vi "save_to_binary_file.vi"(4 "offset (0)":dbl, 5 "prepend array size?":bool, 6 "multiplication factor (1)":dbl=1.0, 7 "force format?":T1, 8 "error in (no error)":errorcluster, 9 "byte order (0:big-endian, network order)":T2(ring)=enum."little-endian", 10 "Path":path, 11 "Image in":refnum<class "Image.lvclass">) -> (0 "error out":errorcluster, 3 "Image out":refnum<class "Image.lvclass">)   [LabVIEW 2010, in "Image.lvclass"]
uses:
  Image.lvclass
  target_format_enum.ctl
  storage_mode.ctl
  error_codes_ring.ctl
  ErrorController/ErrorController/class_data.vi
  ErrorController/ErrorController/ErrorController.lvclass
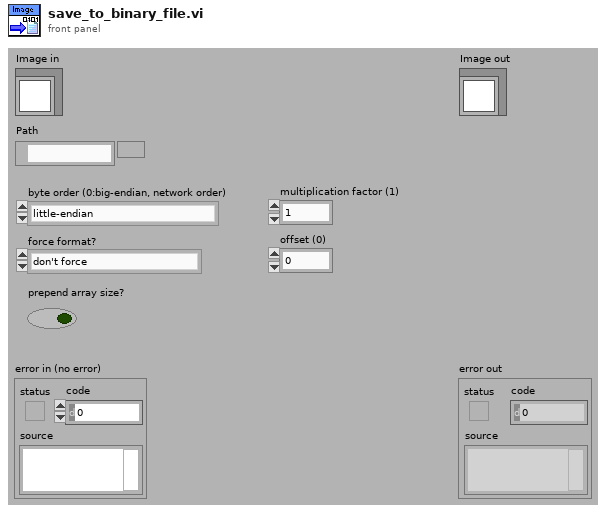
[diagram p1: front panel]
types:
  T1 = typedef "target_format_enum.ctl" = enum16{"don't force", "uint8", "uint16", "int16", "uint32", "int32", "single float"}
  T2 = enum16{"big-endian, network order", "native, host order", "little-endian"}
  T3 = typedef "Image.lvclass/storage_mode.ctl" = enum16{"RAM", "disk"}
  T4 = typedef "Image Type" = u32
  T5 = typedef "IMAQ Image.ctl" = refnum<image>
  T6 = typedef "Color (U64)" = cluster{"Plane 3 (Blue)":u16, "Plane 2 (Green)":u16, "Plane 1 (Red)":u16, "Plane 4 (alpha)":u16}
  T7 = typedef "Image.lvclass/error_codes_ring.ctl" = u16
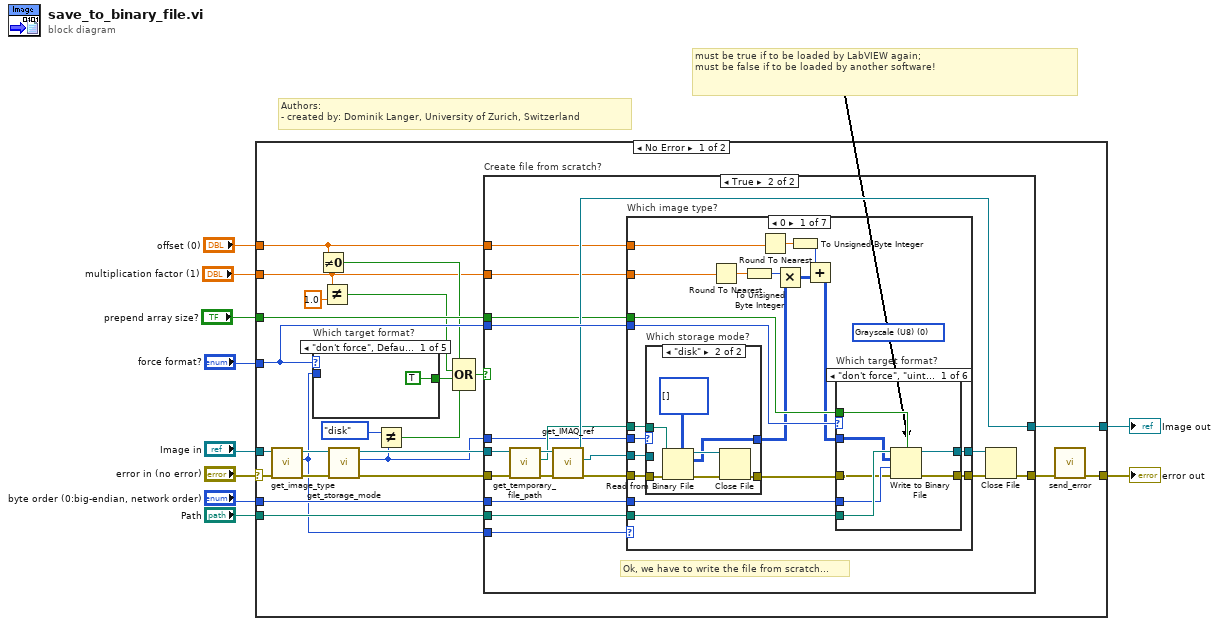
[diagram p0: block diagram]
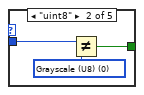
[diagram p2: hidden frame]
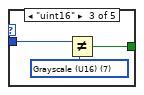
[diagram p3: hidden frame]
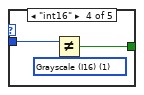
[diagram p4: hidden frame]
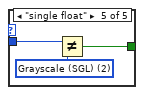
[diagram p5: hidden frame]
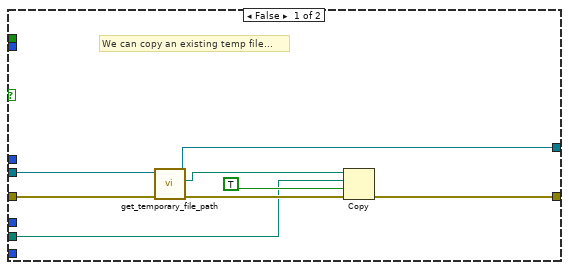
[diagram p6: hidden frame]
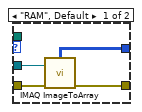
[diagram p7: hidden frame]
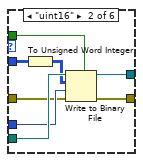
[diagram p8: hidden frame]
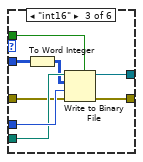
[diagram p9: hidden frame]
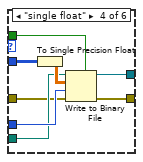
[diagram p10: hidden frame]
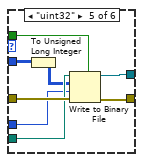
[diagram p11: hidden frame]
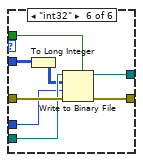
[diagram p12: hidden frame]
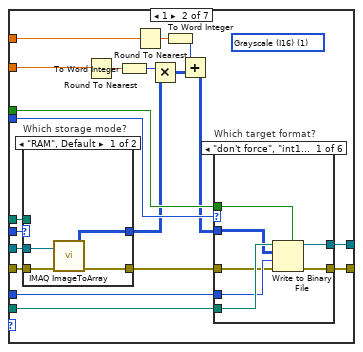
[diagram p13: hidden frame]
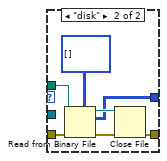
[diagram p14: hidden frame]
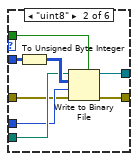
[diagram p15: hidden frame]
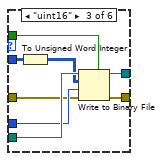
[diagram p16: hidden frame]
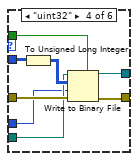
[diagram p17: hidden frame]
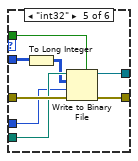
[diagram p18: hidden frame]
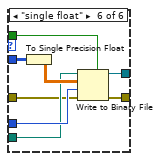
[diagram p19: hidden frame]
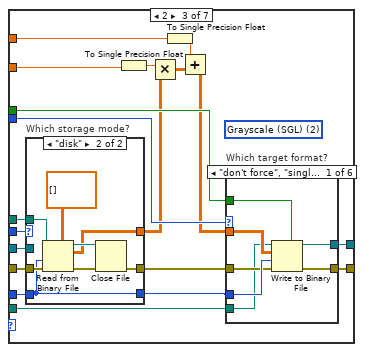
[diagram p20: hidden frame]
diagram:
  # "must be true if to be loaded by LabVIEW again;\nmust be false if to be loaded by another software!"
  # "Authors: \n- created by: Dominik Langer, University of Zurich, Switzerland"
  n1 = case shown="No Error" "error in (no error)" {
    selector: "error in (no error)" -> [w34 w414]
    tunnel: [w12 w414] -> w5
    tunnel: [w25 w413] -> w4
    tunnel: "Image in" -> [w33 w413]
    tunnel: "Path" -> [w26 _]
    tunnel: "byte order (0:big-endian, network order)" -> [w27 _]
    tunnel: "force format?" -> [w23 _]
    tunnel: "prepend array size?" -> [w22 _]
    tunnel: "offset (0)" -> [w14 _]
    tunnel: "multiplication factor (1)" -> [w13 _]
    frame No Error {
      n2 = call-dynamic "get_image_type.vi"("error in (no error)"=w34, "Image.lvclass in"=w33) -> ("error out"=w32:errorcluster, "Image Type"=w24:T4, "Image.lvclass out"=w31:refnum<class "Image.lvclass">)  [unwired: 6 in, 1 out]
      n3 = case "Which target format?" shown="\"don't force\", Default" w23 {
        tunnel: w24 -> [_ w38 w41 w44 w47]
        tunnel: [TRUE w36 w39 w42 w45] -> w16
        frame "don't force", Default {
        }
        frame "uint8" {
          w37 = T4 0 items=["Grayscale (U8)", "Grayscale (I16)", "Grayscale (SGL)", "Complex (CSG)", "RGB (U32)", "HSL (U32)", "RGB (U64)", "Grayscale (U16)"] ("y")
          n4 = Not Equal?(x=w38, y=w37) -> (x != y?=w36:bool)
        }
        frame "uint16" {
          w40 = T4 7 items=["Grayscale (U8)", "Grayscale (I16)", "Grayscale (SGL)", "Complex (CSG)", "RGB (U32)", "HSL (U32)", "RGB (U64)", "Grayscale (U16)"] ("y")
          n5 = Not Equal?(x=w41, y=w40) -> (x != y?=w39:bool)
        }
        frame "int16" {
          w43 = T4 1 items=["Grayscale (U8)", "Grayscale (I16)", "Grayscale (SGL)", "Complex (CSG)", "RGB (U32)", "HSL (U32)", "RGB (U64)", "Grayscale (U16)"] ("y")
          n6 = Not Equal?(x=w44, y=w43) -> (x != y?=w42:bool)
        }
        frame "single float" {
          w46 = T4 2 items=["Grayscale (U8)", "Grayscale (I16)", "Grayscale (SGL)", "Complex (CSG)", "RGB (U32)", "HSL (U32)", "RGB (U64)", "Grayscale (U16)"] ("y")
          n7 = Not Equal?(x=w47, y=w46) -> (x != y?=w45:bool)
        }
      }
      n8 = Not Equal To 0?(x=w14) -> (x != 0?=w20:bool)
      n9 = Not Equal?(x=w13, y=1.0) -> (x != y?=w15:bool)
      n10 = call-dynamic "get_storage_mode.vi"("error in (no error)"=w32, "Image.lvclass in"=w31) -> ("error out"=w29:errorcluster, "storage mode"=w19:T3, "Image.lvclass out"=w28:refnum<class "Image.lvclass">)  [unwired: 7 out]
      n11 = Not Equal?(x=storage_mode."disk", y=w19) -> (x != y?=w18:bool)
      n12 = Compound Arithmetic op=OR(w20, w15, w16, w18) -> (w17:bool)
      n13 = case "Create file from scratch?" shown="True" w17 {
        tunnel: w29 -> [w52 w66]
        tunnel: [w51 w62] -> w11
        tunnel: w28 -> [w49 w65]
        tunnel: w27 -> [_ w70]
        tunnel: w26 -> [w50 w69]
        tunnel: [w48 w61] -> w25
        tunnel: w24 -> [_ w68]
        tunnel: w23 -> [_ w67]
        tunnel: w22 -> [_ w59]
        tunnel: w19 -> [_ w58]
        tunnel: w14 -> [_ w57]
        tunnel: w13 -> [_ w56]
        frame False {
          # "We can copy an existing temp file..."
          n14 = call-dynamic "get_temporary_file_path.vi"("error in (no error)"=w52, "Image.lvclass in"=w49) -> ("error out"=w55:errorcluster, "temporary file path"=w54:path, "Image.lvclass out"=w48:refnum<class "Image.lvclass">)  [unwired: 7 out]
          n15 = Copy(8:w55, 9:TRUE ("overwrite (F)"), 10:w50, 11:w54) -> (0:w51:errorcluster)  [unwired: 3 out]
        }
        frame True {
          # "Ok, we have to write the file from scratch..."
          n16 = call-dynamic "get_temporary_file_path.vi"("error in (no error)"=w66, "Image.lvclass in"=w65) -> ("error out"=w64:errorcluster, "temporary file path"=w60:path, "Image.lvclass out"=w63:refnum<class "Image.lvclass">)  [unwired: 7 out]
          n17 = call-dynamic "get_IMAQ_ref.vi"("error in (no error)"=w64, "Image.lvclass in"=w63) -> ("error out"=w74:errorcluster, "Image"=w73:T5, "Image.lvclass out"=w61:refnum<class "Image.lvclass">)  [unwired: 7 out]
          n18 = case "Which image type?" shown="0" w68 {
            tunnel: [w94 w172 w245 w315 w325 w347 w406] -> w72
            tunnel: w73 -> [w87 w164 w248 w317 w324 w339 _]
            tunnel: w74 -> [w89 w167 w249 w318 w326 w342 w407]
            tunnel: [w93 w171 w244 w313 w322 w346 _] -> w71
            tunnel: w69 -> [w92 w169 w246 w312 w321 w343 _]
            tunnel: w70 -> [w91 w170 w241 w311 w320 w344 _]
            tunnel: w67 -> [w90 w168 w243 _ _ w345 _]
            tunnel: w60 -> [w86 w165 w242 _ _ w340 _]
            tunnel: w59 -> [w85 w163 w239 w310 w319 w338 _]
            tunnel: w58 -> [w84 w162 w238 _ _ w337 _]
            tunnel: w57 -> [w77 w158 w231 _ _ w331 _]
            tunnel: w56 -> [w78 w160 w234 _ _ w332 _]
            frame 0 {
              (unwired) T4 0 items=["Grayscale (U8)", "Grayscale (I16)", "Grayscale (SGL)", "Complex (CSG)", "RGB (U32)", "HSL (U32)", "RGB (U64)", "Grayscale (U16)"] ("Image Type")
              n19 = case "Which storage mode?" shown="\"disk\"" w84 {
                tunnel: w89 -> [w98 w103]
                tunnel: w87 -> [w97 _]
                tunnel: [w96 w102] -> w88
                tunnel: [w95 w100] -> w75
                tunnel: w86 -> [_ w101]
                frame "RAM", Default {
                  n20 = call "IMAQ ImageToArray"("error in (no error)"=w98, "Image"=w97) -> ("error out"=w96:errorcluster, "Image Pixels (U8)"=w95:u8[][])  [unwired: 1 in, 4 out]
                }
                frame "disk" {
                  n21 = Read from Binary File(5:u8[][] [], 8:w103, 11:w101) -> (0:w105:errorcluster, 2:w100:u8[][], 3:w104:refnum<file>)  [unwired: 1 in, 3 out]
                  n22 = Close File(refnum=w104, error in=w105) -> (error out=w102:errorcluster)  [unwired: 1 out]
                }
              }
              n23 = Round To Nearest(number=w78) -> (nearest integer value=w82:dbl)
              n24 = To Unsigned Byte Integer(number=w82) -> (unsigned 8bit integer=w83:u8)
              n25 = Round To Nearest(number=w77) -> (nearest integer value=w81:dbl)
              n26 = Multiply(x=w83, y=w75) -> (x*y=w79:u8[][])
              n27 = To Unsigned Byte Integer(number=w81) -> (unsigned 8bit integer=w80:u8)
              n28 = Add(x=w80, y=w79) -> (x+y=w76:u8[][])
              n29 = case "Which target format?" shown="\"don't force\", \"uint8\", Default" w90 {
                tunnel: [w112 w117 w128 w135 w139 w151] -> w94
                tunnel: w88 -> [w107 w114 w123 w130 w144 w152]
                tunnel: [w111 w116 w125 w134 w138 w150] -> w93
                tunnel: w92 -> [w110 w120 w126 w132 w141 w147]
                tunnel: w91 -> [w109 w119 w127 w133 w140 w146]
                tunnel: w76 -> [w108 w115 w122 w131 w143 w149]
                tunnel: w85 -> [w106 w113 w121 w129 w142 w148]
                frame "don't force", "uint8", Default {
                  n30 = Write to Binary File(file (use dialog)=w110, data=w108, error in=w107, 5:w106, 9:w109) -> (refnum out=w111:refnum<file>, error out=w112:errorcluster)  [unwired: 2 out]
                }
                frame "uint16" {
                  n31 = To Unsigned Word Integer(number=w115) -> (unsigned 16bit integer=w118:u16[][])
                  n32 = Write to Binary File(file (use dialog)=w120, data=w118, error in=w114, 5:w113, 9:w119) -> (refnum out=w116:refnum<file>, error out=w117:errorcluster)  [unwired: 2 out]
                }
                frame "int16" {
                  n33 = To Word Integer(number=w122) -> (16bit integer=w124:i16[][])
                  n34 = Write to Binary File(file (use dialog)=w126, data=w124, error in=w123, 5:w121, 9:w127) -> (refnum out=w125:refnum<file>, error out=w128:errorcluster)  [unwired: 2 out]
                }
                frame "single float" {
                  n35 = To Single Precision Float(number=w131) -> (single precision float=w136:sgl[][])
                  n36 = Write to Binary File(file (use dialog)=w132, data=w136, error in=w130, 5:w129, 9:w133) -> (refnum out=w134:refnum<file>, error out=w135:errorcluster)  [unwired: 2 out]
                }
                frame "uint32" {
                  n37 = To Unsigned Long Integer(number=w143) -> (unsigned 32bit integer=w137:u32[][])
                  n38 = Write to Binary File(file (use dialog)=w141, data=w137, error in=w144, 5:w142, 9:w140) -> (refnum out=w138:refnum<file>, error out=w139:errorcluster)  [unwired: 2 out]
                }
                frame "int32" {
                  n39 = To Long Integer(number=w149) -> (32bit integer=w145:i32[][])
                  n40 = Write to Binary File(file (use dialog)=w147, data=w145, error in=w152, 5:w148, 9:w146) -> (refnum out=w150:refnum<file>, error out=w151:errorcluster)  [unwired: 2 out]
                }
              }
            }
            frame 1 {
              (unwired) T4 1 items=["Grayscale (U8)", "Grayscale (I16)", "Grayscale (SGL)", "Complex (CSG)", "RGB (U32)", "HSL (U32)", "RGB (U64)", "Grayscale (U16)"] ("Image Type")
              n41 = case "Which storage mode?" shown="\"RAM\", Default" w162 {
                tunnel: w167 -> [w176 w181]
                tunnel: w164 -> [w175 _]
                tunnel: [w174 w180] -> w166
                tunnel: [w173 w178] -> w153
                tunnel: w165 -> [_ w179]
                frame "RAM", Default {
                  n42 = call "IMAQ ImageToArray"("error in (no error)"=w176, "Image"=w175) -> ("error out"=w174:errorcluster, "Image Pixels (I16)"=w173:i16[][])  [unwired: 1 in, 4 out]
                }
                frame "disk" {
                  n43 = Read from Binary File(5:i16[][] [], 8:w181, 11:w179) -> (0:w183:errorcluster, 2:w178:i16[][], 3:w182:refnum<file>)  [unwired: 1 in, 3 out]
                  n44 = Close File(refnum=w182, error in=w183) -> (error out=w180:errorcluster)  [unwired: 1 out]
                }
              }
              n45 = Round To Nearest(number=w160) -> (nearest integer value=w159:dbl)
              n46 = To Word Integer(number=w159) -> (16bit integer=w161:i16)
              n47 = Round To Nearest(number=w158) -> (nearest integer value=w157:dbl)
              n48 = Multiply(x=w161, y=w153) -> (x*y=w155:i16[][])
              n49 = To Word Integer(number=w157) -> (16bit integer=w156:i16)
              n50 = Add(x=w156, y=w155) -> (x+y=w154:i16[][])
              n51 = case "Which target format?" shown="\"don't force\", \"int16\", Default" w168 {
                tunnel: [w190 w197 w203 w213 w221 w229] -> w172
                tunnel: w166 -> [w186 w193 w201 w214 w222 w225]
                tunnel: [w189 w196 w202 w212 w220 w228] -> w171
                tunnel: w169 -> [w188 w195 w206 w208 w218 w226]
                tunnel: w170 -> [w187 w194 w205 w207 w217 w227]
                tunnel: w154 -> [w185 w192 w200 w210 w215 w224]
                tunnel: w163 -> [w184 w191 w199 w209 w219 w223]
                frame "don't force", "int16", Default {
                  n52 = Write to Binary File(file (use dialog)=w188, data=w185, error in=w186, 5:w184, 9:w187) -> (refnum out=w189:refnum<file>, error out=w190:errorcluster)  [unwired: 2 out]
                }
                frame "uint8" {
                  n53 = To Unsigned Byte Integer(number=w192) -> (unsigned 8bit integer=w198:u8[][])
                  n54 = Write to Binary File(file (use dialog)=w195, data=w198, error in=w193, 5:w191, 9:w194) -> (refnum out=w196:refnum<file>, error out=w197:errorcluster)  [unwired: 2 out]
                }
                frame "uint16" {
                  n55 = To Unsigned Word Integer(number=w200) -> (unsigned 16bit integer=w204:u16[][])
                  n56 = Write to Binary File(file (use dialog)=w206, data=w204, error in=w201, 5:w199, 9:w205) -> (refnum out=w202:refnum<file>, error out=w203:errorcluster)  [unwired: 2 out]
                }
                frame "uint32" {
                  n57 = To Unsigned Long Integer(number=w210) -> (unsigned 32bit integer=w211:u32[][])
                  n58 = Write to Binary File(file (use dialog)=w208, data=w211, error in=w214, 5:w209, 9:w207) -> (refnum out=w212:refnum<file>, error out=w213:errorcluster)  [unwired: 2 out]
                }
                frame "int32" {
                  n59 = To Long Integer(number=w215) -> (32bit integer=w216:i32[][])
                  n60 = Write to Binary File(file (use dialog)=w218, data=w216, error in=w222, 5:w219, 9:w217) -> (refnum out=w220:refnum<file>, error out=w221:errorcluster)  [unwired: 2 out]
                }
                frame "single float" {
                  n61 = To Single Precision Float(number=w224) -> (single precision float=w230:sgl[][])
                  n62 = Write to Binary File(file (use dialog)=w226, data=w230, error in=w225, 5:w223, 9:w227) -> (refnum out=w228:refnum<file>, error out=w229:errorcluster)  [unwired: 2 out]
                }
              }
            }
            frame 2 {
              (unwired) T4 2 items=["Grayscale (U8)", "Grayscale (I16)", "Grayscale (SGL)", "Complex (CSG)", "RGB (U32)", "HSL (U32)", "RGB (U64)", "Grayscale (U16)"] ("Image Type")
              n63 = case "Which storage mode?" shown="\"disk\"" w238 {
                tunnel: w249 -> [w254 w260]
                tunnel: w248 -> [w253 _]
                tunnel: [w252 w259] -> w247
                tunnel: [w251 w255] -> w232
                tunnel: w242 -> [_ w258]
                tunnel: w241 -> [w250 w256]
                tunnel: [w250 w256] -> w240
                frame "RAM", Default {
                  n64 = call "IMAQ ImageToArray"("error in (no error)"=w254, "Image"=w253) -> ("Image Pixels (Float)"=w251:sgl[][], "error out"=w252:errorcluster)  [unwired: 1 in, 4 out]
                }
                frame "disk" {
                  n65 = Read from Binary File(5:sgl[][] [], 8:w260, 9:w256, 11:w258) -> (0:w262:errorcluster, 2:w255:sgl[][], 3:w261:refnum<file>)  [unwired: 1 in, 2 out]
                  n66 = Close File(refnum=w261, error in=w262) -> (error out=w259:errorcluster)  [unwired: 1 out]
                }
              }
              n67 = To Single Precision Float(number=w234) -> (single precision float=w237:sgl)
              n68 = Multiply(x=w237, y=w232) -> (x*y=w235:sgl[][])
              n69 = To Single Precision Float(number=w231) -> (single precision float=w236:sgl)
              n70 = Add(x=w236, y=w235) -> (x+y=w233:sgl[][])
              n71 = case "Which target format?" shown="\"don't force\", \"single float\", Default" w243 {
                tunnel: [w269 w272 w284 w293 w298 w306] -> w245
                tunnel: w247 -> [w265 w274 w281 w288 w301 w307]
                tunnel: [w268 w271 w283 w290 w300 w305] -> w244
                tunnel: w246 -> [w264 w275 w280 w291 w294 w303]
                tunnel: w240 -> [w267 w276 w285 w292 w295 w302]
                tunnel: w233 -> [w266 w273 w282 w287 w297 w308]
                tunnel: w239 -> [w263 w270 w278 w286 w299 w304]
                frame "don't force", "single float", Default {
                  n72 = Write to Binary File(file (use dialog)=w264, data=w266, error in=w265, 5:w263, 9:w267) -> (refnum out=w268:refnum<file>, error out=w269:errorcluster)  [unwired: 2 out]
                }
                frame "uint8" {
                  n73 = To Unsigned Byte Integer(number=w273) -> (unsigned 8bit integer=w277:u8[][])
                  n74 = Write to Binary File(file (use dialog)=w275, data=w277, error in=w274, 5:w270, 9:w276) -> (refnum out=w271:refnum<file>, error out=w272:errorcluster)  [unwired: 2 out]
                }
                frame "uint16" {
                  n75 = To Unsigned Word Integer(number=w282) -> (unsigned 16bit integer=w279:u16[][])
                  n76 = Write to Binary File(file (use dialog)=w280, data=w279, error in=w281, 5:w278, 9:w285) -> (refnum out=w283:refnum<file>, error out=w284:errorcluster)  [unwired: 2 out]
                }
                frame "int16" {
                  n77 = To Word Integer(number=w287) -> (16bit integer=w289:i16[][])
                  n78 = Write to Binary File(file (use dialog)=w291, data=w289, error in=w288, 5:w286, 9:w292) -> (refnum out=w290:refnum<file>, error out=w293:errorcluster)  [unwired: 2 out]
                }
                frame "uint32" {
                  n79 = To Unsigned Long Integer(number=w297) -> (unsigned 32bit integer=w296:u32[][])
                  n80 = Write to Binary File(file (use dialog)=w294, data=w296, error in=w301, 5:w299, 9:w295) -> (refnum out=w300:refnum<file>, error out=w298:errorcluster)  [unwired: 2 out]
                }
                frame "int32" {
                  n81 = To Long Integer(number=w308) -> (32bit integer=w309:i32[][])
                  n82 = Write to Binary File(file (use dialog)=w303, data=w309, error in=w307, 5:w304, 9:w302) -> (refnum out=w305:refnum<file>, error out=w306:errorcluster)  [unwired: 2 out]
                }
              }
            }
            frame 4 {
              (unwired) T4 4 items=["Grayscale (U8)", "Grayscale (I16)", "Grayscale (SGL)", "Complex (CSG)", "RGB (U32)", "HSL (U32)", "RGB (U64)", "Grayscale (U16)"] ("Image Type")
              # "Target file format will be omitted..."
              n83 = call "IMAQ ColorImageToArray"("Image"=w317, "error in (no error)"=w318) -> ("Image Pixels (U32)"=w314:u32[][], "error out"=w316:errorcluster)  [unwired: 1 in, 2 out]
              n84 = Write to Binary File(file (use dialog)=w312, data=w314, error in=w316, 5:w310, 9:w311) -> (refnum out=w313:refnum<file>, error out=w315:errorcluster)  [unwired: 2 out]
            }
            frame 6 {
              (unwired) T4 6 items=["Grayscale (U8)", "Grayscale (I16)", "Grayscale (SGL)", "Complex (CSG)", "RGB (U32)", "HSL (U32)", "RGB (U64)", "Grayscale (U16)"] ("Image Type")
              # "Target file format will be omitted..."
              n85 = call "IMAQ ColorImageToArray"("Image"=w324, "error in (no error)"=w326) -> ("error out"=w327:errorcluster, "Image Pixels (U64)"=w323:T6[][])  [unwired: 1 in, 2 out]
              n86 = Write to Binary File(file (use dialog)=w321, data=w323, error in=w327, 5:w319, 9:w320) -> (refnum out=w322:refnum<file>, error out=w325:errorcluster)  [unwired: 2 out]
            }
            frame 7 {
              (unwired) T4 7 items=["Grayscale (U8)", "Grayscale (I16)", "Grayscale (SGL)", "Complex (CSG)", "RGB (U32)", "HSL (U32)", "RGB (U64)", "Grayscale (U16)"] ("Image Type")
              n87 = case "Which storage mode?" shown="\"RAM\", Default" w337 {
                tunnel: w342 -> [w351 w356]
                tunnel: w339 -> [w350 _]
                tunnel: [w349 w355] -> w341
                tunnel: [w348 w353] -> w328
                tunnel: w340 -> [_ w354]
                frame "RAM", Default {
                  n88 = call "IMAQ ImageToArray"("error in (no error)"=w351, "Image"=w350) -> ("Image Pixels (U16)"=w348:u16[][], "error out"=w349:errorcluster)  [unwired: 1 in, 4 out]
                }
                frame "disk" {
                  n89 = Read from Binary File(5:u16[][] [], 8:w356, 11:w354) -> (0:w358:errorcluster, 2:w353:u16[][], 3:w357:refnum<file>)  [unwired: 1 in, 3 out]
                  n90 = Close File(refnum=w357, error in=w358) -> (error out=w355:errorcluster)  [unwired: 1 out]
                }
              }
              n91 = Round To Nearest(number=w332) -> (nearest integer value=w335:dbl)
              n92 = To Unsigned Word Integer(number=w335) -> (unsigned 16bit integer=w336:u16)
              n93 = Round To Nearest(number=w331) -> (nearest integer value=w330:dbl)
              n94 = Multiply(x=w336, y=w328) -> (x*y=w333:u16[][])
              n95 = To Unsigned Word Integer(number=w330) -> (unsigned 16bit integer=w334:u16)
              n96 = Add(x=w334, y=w333) -> (x+y=w329:u16[][])
              n97 = case "Which target format?" shown="\"single float\"" w345 {
                tunnel: [w365 w370 w381 w388 w396 w404] -> w347
                tunnel: w341 -> [w360 w367 w376 w389 w397 w399]
                tunnel: [w364 w369 w378 w387 w395 w403] -> w346
                tunnel: w343 -> [w363 w373 w379 w384 w390 w401]
                tunnel: w344 -> [w362 w372 w380 w383 w391 w402]
                tunnel: w329 -> [w361 w368 w375 w386 w393 w400]
                tunnel: w338 -> [w359 w366 w374 w382 w392 w398]
                frame "don't force", "uint16", Default {
                  n98 = Write to Binary File(file (use dialog)=w363, data=w361, error in=w360, 5:w359, 9:w362) -> (refnum out=w364:refnum<file>, error out=w365:errorcluster)  [unwired: 2 out]
                }
                frame "uint8" {
                  n99 = To Unsigned Byte Integer(number=w368) -> (unsigned 8bit integer=w371:u8[][])
                  n100 = Write to Binary File(file (use dialog)=w373, data=w371, error in=w367, 5:w366, 9:w372) -> (refnum out=w369:refnum<file>, error out=w370:errorcluster)  [unwired: 2 out]
                }
                frame "int16" {
                  n101 = To Word Integer(number=w375) -> (16bit integer=w377:i16[][])
                  n102 = Write to Binary File(file (use dialog)=w379, data=w377, error in=w376, 5:w374, 9:w380) -> (refnum out=w378:refnum<file>, error out=w381:errorcluster)  [unwired: 2 out]
                }
                frame "uint32" {
                  n103 = To Unsigned Long Integer(number=w386) -> (unsigned 32bit integer=w385:u32[][])
                  n104 = Write to Binary File(file (use dialog)=w384, data=w385, error in=w389, 5:w382, 9:w383) -> (refnum out=w387:refnum<file>, error out=w388:errorcluster)  [unwired: 2 out]
                }
                frame "int32" {
                  n105 = To Long Integer(number=w393) -> (32bit integer=w394:i32[][])
                  n106 = Write to Binary File(file (use dialog)=w390, data=w394, error in=w397, 5:w392, 9:w391) -> (refnum out=w395:refnum<file>, error out=w396:errorcluster)  [unwired: 2 out]
                }
                frame "single float" {
                  n107 = To Single Precision Float(number=w400) -> (single precision float=w405:sgl[][])
                  n108 = Write to Binary File(file (use dialog)=w401, data=w405, error in=w399, 5:w398, 9:w402) -> (refnum out=w403:refnum<file>, error out=w404:errorcluster)  [unwired: 2 out]
                }
              }
            }
            frame Default {
              n109 = case shown="No Error" w407 {
                selector: w407 -> [_ w412]
                tunnel: [w411 w412] -> w406
                frame No Error {
                  w409 = T7 5000 items=["Image type not supported"=5000] ("Ring")
                  n110 = To Long Integer(number=w409) -> (32bit integer=w408:i32)
                  n111 = call <userlib>:"Build Error Cluster__ogtk.vi"("String to Prepend to source (\"\")"="Image:clear.vi - image type not supported" ("String to Prepend to source (\"\")"), "code"=w408) -> ("error out"=w411:errorcluster)
                }
                frame Error {
                }
              }
            }
          }
          n112 = Close File(refnum=w71, error in=w72) -> (error out=w62:errorcluster)  [unwired: 1 out]
        }
      }
      n113 = call "send_error.vi"("error in (no error)"=w11) -> ("error out"=w12:errorcluster)  [unwired: 10 in]
    }
    frame Error {
    }
  }
  "error out" <- w5
  "Image out" <- w4
